vi "Recurse.vi"(6 "Error":errorcluster, 7 "ConcreteActor":refnum<class "ConcreteActor.lvclass">, 11 "Message":refnum<class "Message.lvclass">) -> (3 "Message":refnum<class "Message.lvclass">, 4 "Error":errorcluster, 5 "ConcreteActor":refnum<class "ConcreteActor.lvclass">)   [LabVIEW 2020, in "_Template.lvlib" / "ActorTemplate.lvlib" / "{{Name}}.lvlib" / "ConcreteActor.lvclass"]
uses:
  ConcreteActor.lvclass
  jettl/jettl/Message/Message.lvclass
  ConcreteActor.lvclass/ConcreteActor.ctl
  jettl/jettl/jettl.lvlib
panel:
  # "This front panel should not be manipulated."
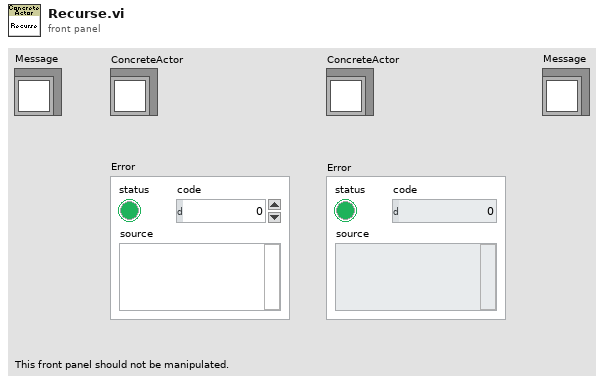
[diagram p1: front panel]
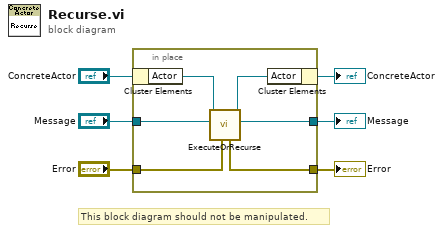
[diagram p0: block diagram]
diagram:
  # "This block diagram should not be manipulated."
  n1 = in-place {
    in-place-border: [w7] -> w6
    in-place-border: "Error" -> [w8]
    in-place-border: "Message" -> [w12]
    in-place-border: [w11] -> w1
    n2 = in-place-cluster #1("ConcreteActor") -> ("Actor"=w10:refnum<class "Actor.lvclass">)
    n3 = call "ExecuteOrRecurse.vi"("Error"=w8, "Message"=w12, "Actor"=w10) -> ("Message"=w11:refnum<class "Message.lvclass">, "Actor"=w9:refnum<class "Actor.lvclass">, "Error"=w7:errorcluster)  [unwired: 6 in]
    n4 = in-place-cluster #1("Actor"=w9) -> (→"ConcreteActor":refnum<class "ConcreteActor.lvclass">)
  }
  "Error" <- w6
  "Message" <- w1
